vi "newTestStandObjRef.vi"(0 "Engine Reference":refnum<k7>, 5 "Sequence File Ref":refnum<k7>, 7 "Variable Name":string="Locals.temp", 11 "error in":errorcluster) -> (4 "Engine Reference (out)":refnum<k7>, 6 "Sequence File (out)":refnum<k7>, 15 "error out":errorcluster)   [LabVIEW 2010]
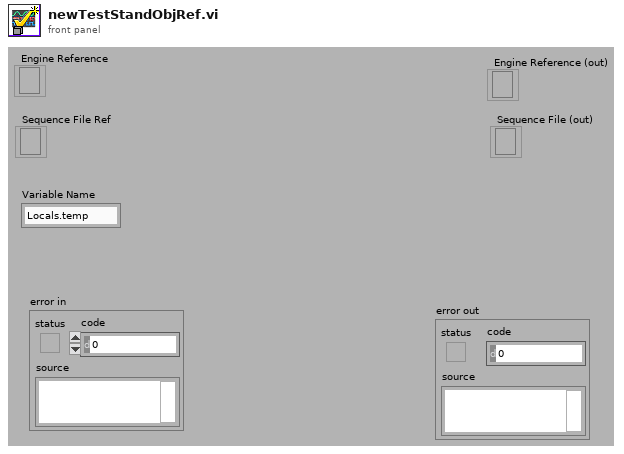
[diagram p1: front panel]
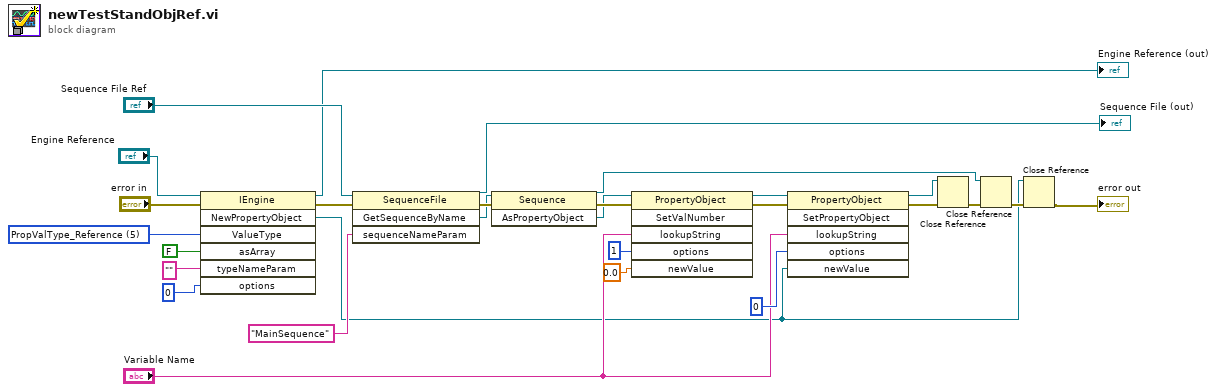
[diagram p0: block diagram]
diagram:
  w24 = 5 items=["PropValType_Container", "PropValType_String", "PropValType_Boolean", "PropValType_Number", "PropValType_NamedType", "PropValType_Reference", "PropValType_Array"] ("ValueType")
  n1 = invoke class="IEngine" method="NewPropertyObject"(reference="Engine Reference", error in="error in", "ValueType"=w24, "asArray"=FALSE, "typeNameParam"="", "options"=0) -> (reference out=→"Engine Reference (out)":refnum<k7>, error out=w5:errorcluster, "NewPropertyObject"=w2:refnum<k7>)  [unwired: 1 in, 4 out]
  n2 = invoke class="SequenceFile" method="GetSequenceByName"(reference="Sequence File Ref", error in=w5, "sequenceNameParam"="MainSequence") -> (reference out=→"Sequence File (out)":refnum<k7>, error out=w12:errorcluster, "GetSequenceByName"=w10:refnum<k7>)  [unwired: 1 in, 1 out]
  n3 = invoke class="Sequence" method="AsPropertyObject"(reference=w10, error in=w12) -> (reference out=w15:refnum<k7>, error out=w7:errorcluster, "AsPropertyObject"=w6:refnum<k7>)  [unwired: 1 in]
  n4 = invoke class="PropertyObject" method="SetValNumber"(reference=w6, error in=w7, "lookupString"="Variable Name", "options"=1, "newValue"=0.0) -> (reference out=w22:refnum<k7>, error out=w17:errorcluster)  [unwired: 1 in, 4 out]
  n5 = invoke class="PropertyObject" method="SetPropertyObject"(reference=w22, error in=w17, "lookupString"="Variable Name", "options"=0, "newValue"=w2) -> (reference out=w18:refnum<k7>, error out=w19:errorcluster)  [unwired: 1 in, 4 out]
  n6 = Close Reference(reference=w18, error in (no error)=w19) -> (error out=w14:errorcluster)
  n7 = Close Reference(reference=w15, error in (no error)=w14) -> (error out=w28:errorcluster)
  n8 = Close Reference(reference=w2, error in (no error)=w28) -> (error out=→"error out":errorcluster)
